vi "Projekt.vi"() -> ()   [LabVIEW 2022 SP3]
doc: "Use this template to build a standard state machine design pattern. Each state executes code and determines which state to transition to. Contrast this design pattern with the User Interface Event Handler pattern, in which code executes in response to user actions. Contrast this design pattern also with the Queued Message Handler pattern, in which each message handling code can queue zero or more new messages.\nNote: This template does not contain the most recent programming guidelines recommended by National Instruments. For a complete, project-based implementation of the Standard State Machine pattern, use the Create Project dialog box instead of this template."
uses:
  Projekt.ctt
  <vilib>/DAQmx/write.llb/DAQmx Write (Digital 1D Bool 1Chan 1Samp).vi
  <vilib>/DAQmx/create/channels.llb/DAQmx Create Channel (DO-Digital Output).vi
  <vilib>/DAQmx/create/channels.llb/DAQmx Create Channel (AI-Voltage-Basic).vi
  <vilib>/DAQmx/create/channels.llb/DAQmx Create Channel (DI-Digital Input).vi
  <vilib>/DAQmx/read.llb/DAQmx Read (Analog DBL 1Chan 1Samp).vi
  <vilib>/DAQmx/read.llb/DAQmx Read (Digital 1D Bool 1Chan 1Samp).vi
panel:
  in  "Buttons":enum32{"Force", "Mass", "Starting height"}(radio)
  in  "LED":tag="Dev3/port0/line0:5"
  in  "Knob":tag="Dev3/ai1"
  in  "Buttons":tag="Dev3/port1/line0:2"
  out "Max S [m]":dbl
  in  "Starting height [m]":dbl
  out "XY Graph":cluster{ext[], ext[]}(graph)
  out "Max H [m]":dbl
  out "V [m/s]":dbl
  in  "Mass [kg]":dbl
  in  "Stop":bool
  in  "Force [n]":dbl
  in  "Angle":dbl(knob) min=0.0 max=90.0 scale=0.0..90.0
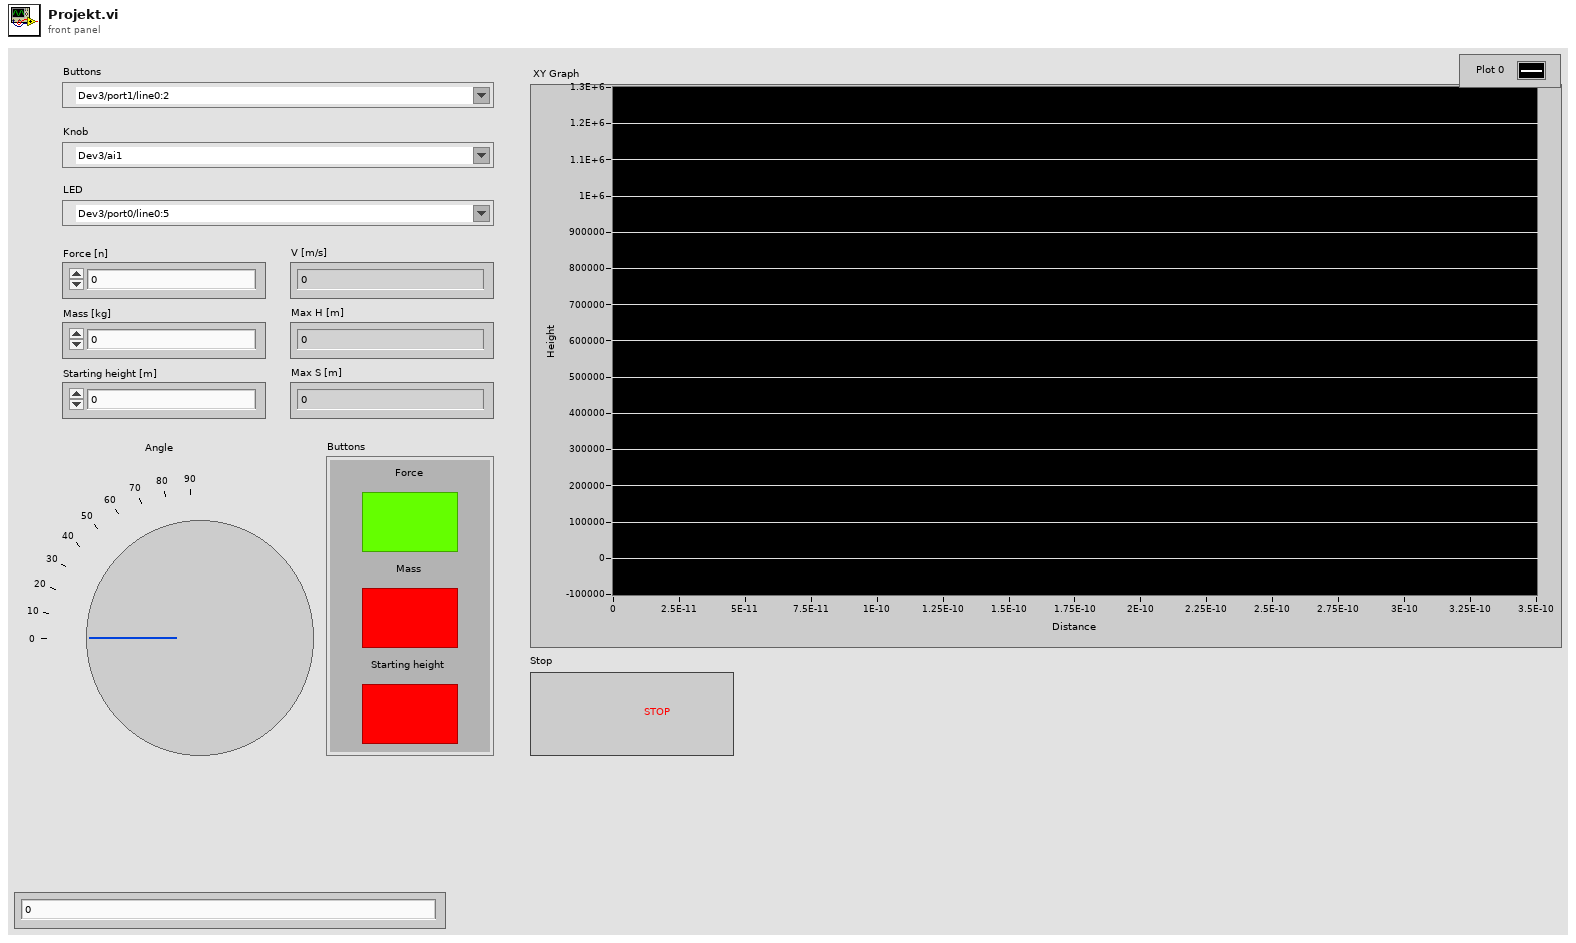
[diagram p1: front panel]
types:
  T1 = typedef "Projekt.ctt" = enum16{"Initialize", "Read", "Simulate", "Stop"}
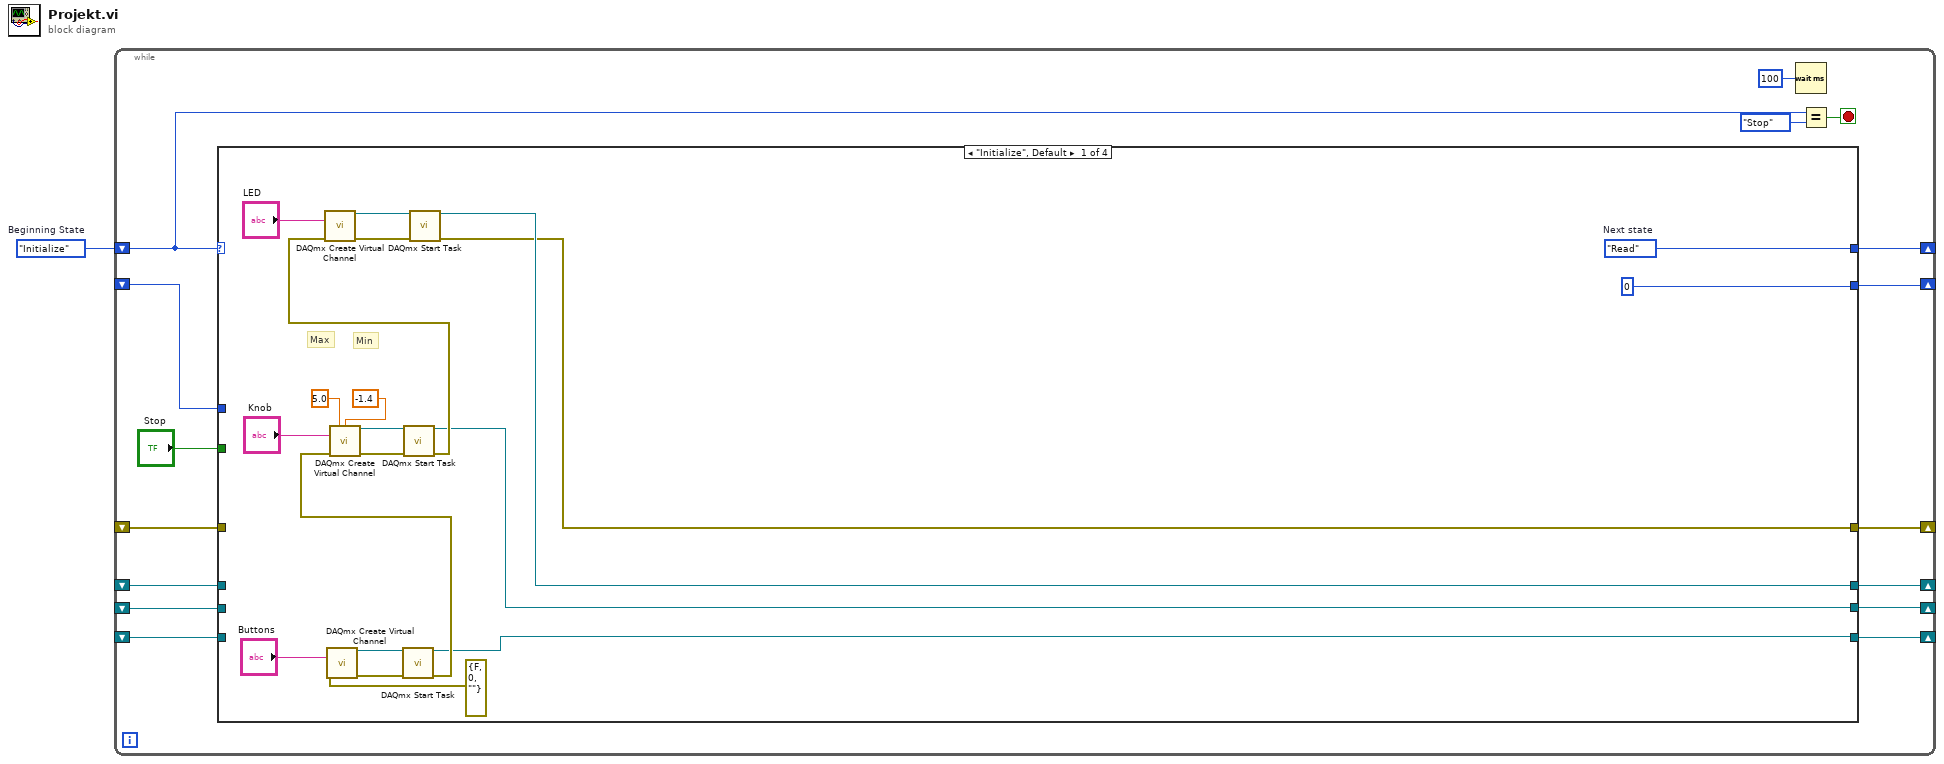
[diagram p0: block diagram]
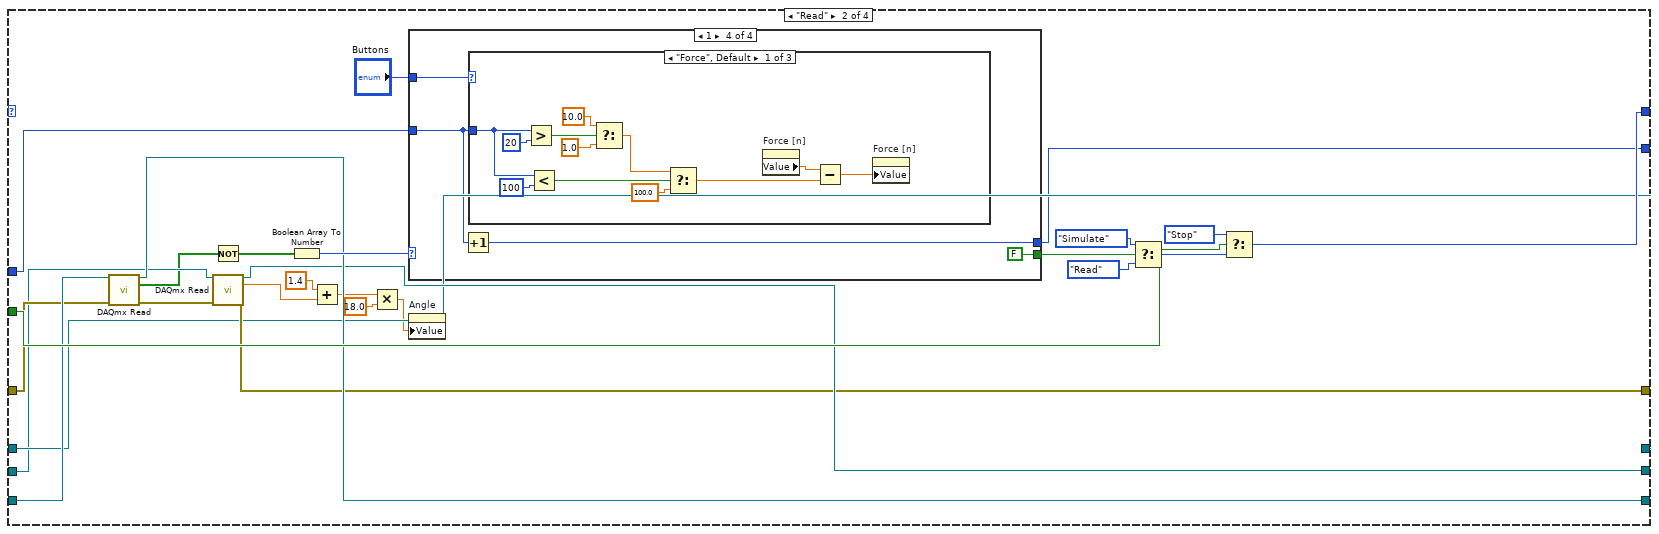
[diagram p2: hidden frame]
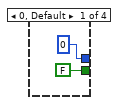
[diagram p3: hidden frame]
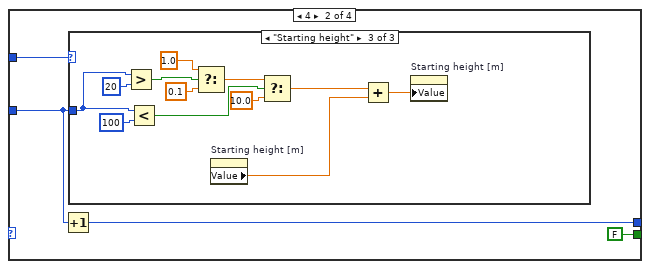
[diagram p4: hidden frame]
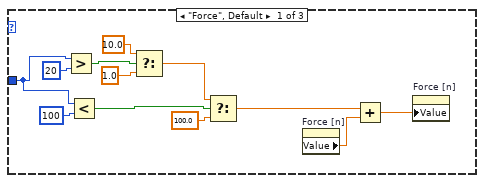
[diagram p5: hidden frame]
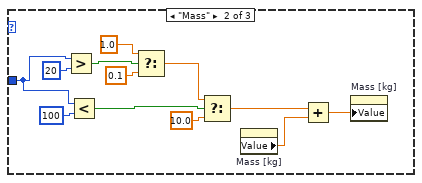
[diagram p6: hidden frame]
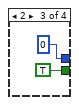
[diagram p7: hidden frame]
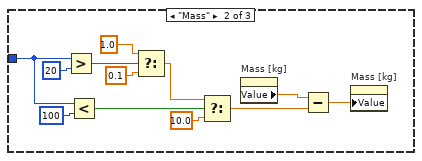
[diagram p8: hidden frame]
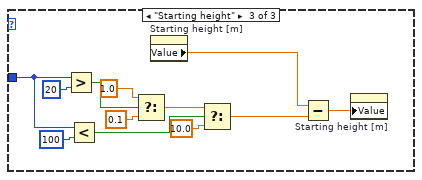
[diagram p9: hidden frame]
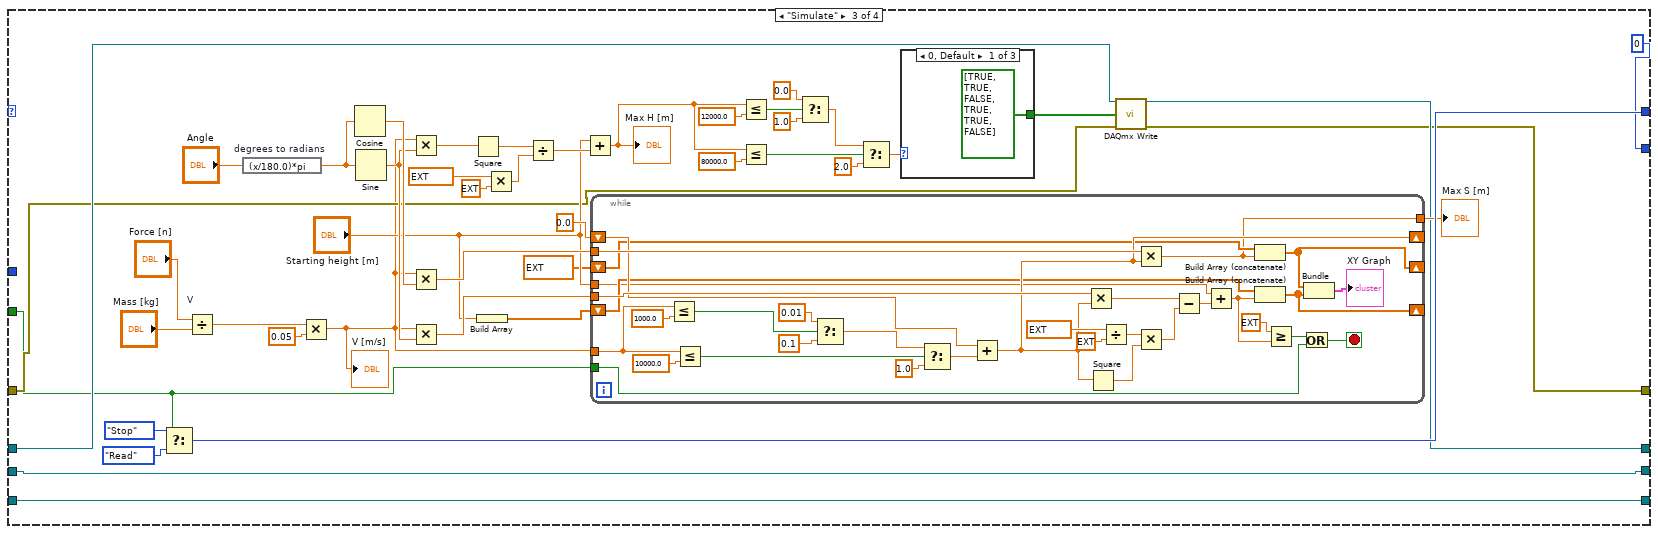
[diagram p10: hidden frame]
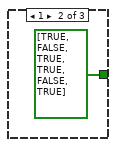
[diagram p11: hidden frame]
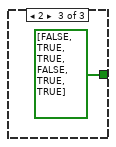
[diagram p12: hidden frame]
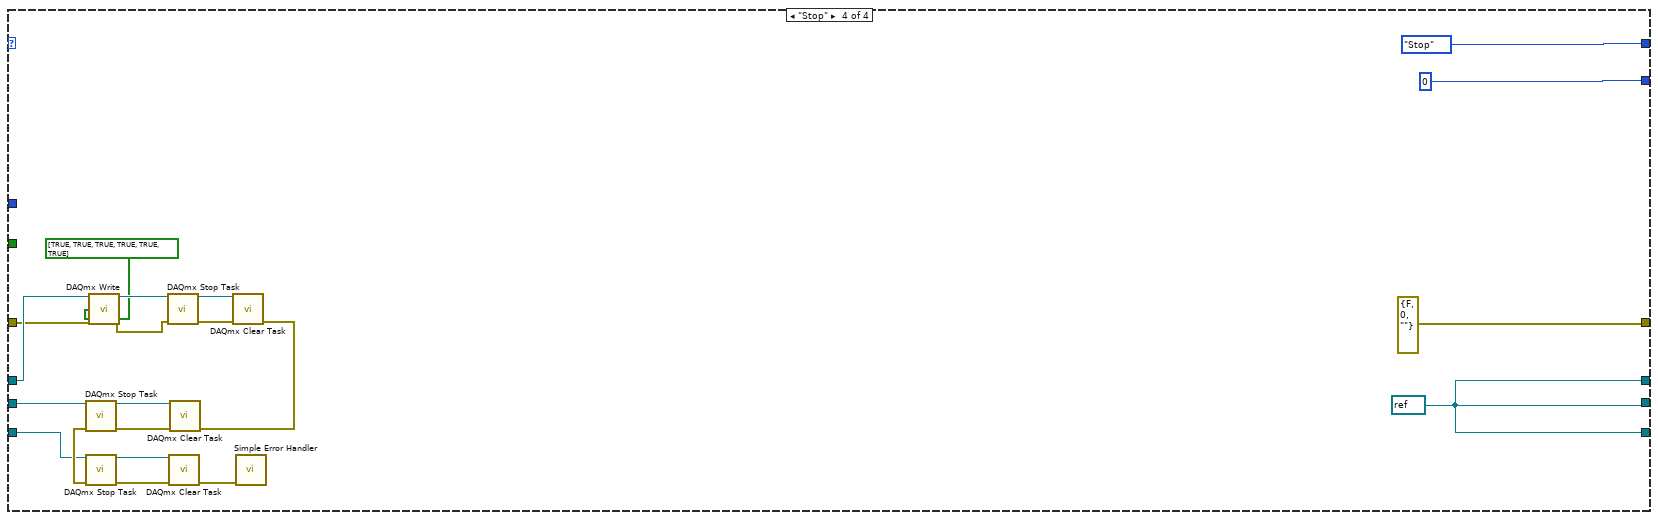
[diagram p13: hidden frame]
diagram:
  w1 = Projekt.ctt."Initialize"  # Beginning State
  n1 = while {
    shift-right: [w14] -> _
    shift-left: w1 -> [w15]
    shift-right: [w11] -> _
    shift-left: _ -> [w5]
    shift-right: [w10] -> _
    shift-left: _ -> [w6]
    shift-right: [w8] -> _
    shift-left: _ -> [w7]
    shift-right: [w9] -> _
    shift-left: _ -> [w4]
    shift-right: [w3] -> _
    shift-left: _ -> [w2]
    stop <- w17 stop-if-true
    n2 = case shown="\"Initialize\", Default" w15 {
      tunnel: [w18 w57 w178 Projekt.ctt."Stop" ("Next State")] -> w14
      tunnel: "Stop" -> [_ w56 w150 _]
      tunnel: w5 -> [_ w55 w168 w237]
      tunnel: [w25 w54 w168 w234] -> w11
      tunnel: [w24 w53 w167 w234] -> w10
      tunnel: [w23 w50 w154 w234] -> w8
      tunnel: [w22 w52 w153 errorcluster {"status"=FALSE, "code"=0, "source"=""} ("error constant")] -> w9
      tunnel: w4 -> [_ w51 w165 w231]
      tunnel: w7 -> [_ w50 w166 w232]
      tunnel: w6 -> [_ w49 w167 w236]
      tunnel: [0 w48 0 0] -> w3
      tunnel: w2 -> [_ w47 _ _]
      frame "Initialize", Default {
        w18 = Projekt.ctt."Read"  # Next state
        # "Max"
        # "Min"
        n3 = call-poly <vilib>:"DAQmx Create Virtual Channel.vi"("lines"="Buttons", "error in"=errorcluster {"status"=FALSE, "code"=0, "source"=""} ("error constant")) -> ("task out"=w37:refnum<k21>, "error out"=w36:errorcluster)  [unwired: 12 in]
        n4 = call <vilib>:"DAQmx Start Task.vi"("task/channels in"=w37, "error in"=w36) -> ("task out"=w25:refnum<k21>, "error out"=w30:errorcluster)  [unwired: 12 in]
        n5 = call-poly <vilib>:"DAQmx Create Virtual Channel.vi"("maximum value"=5.0, "minimum value"=-1.4, "physical channels"="Knob", "error in"=w30) -> ("task out"=w35:refnum<k21>, "error out"=w34:errorcluster)  [unwired: 10 in]
        n6 = call <vilib>:"DAQmx Start Task.vi"("task/channels in"=w35, "error in"=w34) -> ("task out"=w24:refnum<k21>, "error out"=w29:errorcluster)  [unwired: 12 in]
        n7 = call-poly <vilib>:"DAQmx Create Virtual Channel.vi"("lines"="LED", "error in"=w29) -> ("task out"=w33:refnum<k21>, "error out"=w32:errorcluster)  [unwired: 12 in]
        n8 = call <vilib>:"DAQmx Start Task.vi"("task/channels in"=w33, "error in"=w32) -> ("task out"=w23:refnum<k21>, "error out"=w22:errorcluster)  [unwired: 12 in]
      }
      frame "Read" {
        n9 = call-poly <vilib>:"DAQmx Read.vi"("task/channels in"=w55, "error in"=w51) -> ("task out"=w54:refnum<k21>, "data"=w42:bool[], "error out"=w63:errorcluster)  [unwired: 11 in]
        n10 = Not(x=w42) -> (.not. x?=w41:bool[])
        n11 = call-poly <vilib>:"DAQmx Read.vi"("task/channels in"=w49, "error in"=w63) -> ("task out"=w53:refnum<k21>, "data"=w45:dbl, "error out"=w52:errorcluster)  [unwired: 11 in]
        n12 = Boolean Array To Number(Boolean array=w41) -> (number=w60:u32)
        n13 = Add(x=1.4, y=w45) -> (x+y=w43:dbl)
        n14 = Multiply(x=w43, y=18.0) -> (x*y=w46:dbl)
        n15 = case shown="1" w60 {
          tunnel: "Buttons" -> [_ w69 _ w108]
          tunnel: [FALSE FALSE TRUE FALSE] -> w59
          tunnel: [0 w67 0 w109] -> w48
          tunnel: w47 -> [_ w66 _ w110]
          frame 0, Default {
          }
          frame 4 {
            n16 = Increment(x=w66) -> (x+1=w67:i32)
            n17 = case shown="\"Starting height\"" w69 {
              tunnel: w66 -> [w76 w85 w96]
              frame "Force", Default {
                n18 = Greater?(x=w76, y=20) -> (0:w80:bool)
                n19 = Less?(x=w76, y=100) -> (x < y?=w74:bool)
                n20 = Select(t=10.0, s=w80, f=1.0) -> (s? t:f=w77:dbl)
                n21 = Select(t=w77, s=w74, f=100.0) -> (s? t:f=w72:dbl)
                n22 = property on="Force [n]" class="DigNum (strict)"() -> ("Value"=w71:dbl)  [unwired: 2 in, 2 out]
                n23 = Add(x=w72, y=w71) -> (x+y=w70:dbl)
                n24 = property on="Force [n]" class="DigNum (strict)"("Value"=w70) -> ()  [unwired: 2 in, 2 out]
              }
              frame "Mass" {
                n25 = Greater?(x=w85, y=20) -> (0:w92:bool)
                n26 = Less?(x=w85, y=100) -> (x < y?=w87:bool)
                n27 = Select(t=1.0, s=w92, f=0.1) -> (s? t:f=w89:dbl)
                n28 = Select(t=w89, s=w87, f=10.0) -> (s? t:f=w84:dbl)
                n29 = property on="Mass [kg]" class="DigNum (strict)"() -> ("Value"=w83:dbl)  [unwired: 2 in, 2 out]
                n30 = Add(x=w84, y=w83) -> (x+y=w82:dbl)
                n31 = property on="Mass [kg]" class="DigNum (strict)"("Value"=w82) -> ()  [unwired: 2 in, 2 out]
              }
              frame "Starting height" {
                n32 = Greater?(x=w96, y=20) -> (0:w104:bool)
                n33 = Less?(x=w96, y=100) -> (x < y?=w99:bool)
                n34 = Select(t=1.0, s=w104, f=0.1) -> (s? t:f=w101:dbl)
                n35 = property on="Starting height [m]" class="DigNum (strict)"() -> ("Value"=w95:dbl)  [unwired: 2 in, 2 out]
                n36 = Select(t=w101, s=w99, f=10.0) -> (s? t:f=w97:dbl)
                n37 = Add(x=w97, y=w95) -> (x+y=w94:dbl)
                n38 = property on="Starting height [m]" class="DigNum (strict)"("Value"=w94) -> ()  [unwired: 2 in, 2 out]
              }
            }
          }
          frame 2 {
          }
          frame 1 {
            n39 = Increment(x=w110) -> (x+1=w109:i32)
            n40 = case shown="\"Force\", Default" w108 {
              tunnel: w110 -> [w113 w127 w138]
              frame "Force", Default {
                n41 = Greater?(x=w113, y=20) -> (0:w120:bool)
                n42 = Less?(x=w113, y=100) -> (x < y?=w115:bool)
                n43 = Select(t=10.0, s=w120, f=1.0) -> (s? t:f=w117:dbl)
                n44 = Select(t=w117, s=w115, f=100.0) -> (s? t:f=w112:dbl)
                n45 = property on="Force [n]" class="DigNum (strict)"() -> ("Value"=w123:dbl)  [unwired: 2 in, 2 out]
                n46 = Subtract(x=w123, y=w112) -> (x-y=w122:dbl)
                n47 = property on="Force [n]" class="DigNum (strict)"("Value"=w122) -> ()  [unwired: 2 in, 2 out]
              }
              frame "Mass" {
                n48 = Greater?(x=w127, y=20) -> (0:w134:bool)
                n49 = Less?(x=w127, y=100) -> (x < y?=w129:bool)
                n50 = Select(t=1.0, s=w134, f=0.1) -> (s? t:f=w131:dbl)
                n51 = Select(t=w131, s=w129, f=10.0) -> (s? t:f=w124:dbl)
                n52 = property on="Mass [kg]" class="DigNum (strict)"() -> ("Value"=w126:dbl)  [unwired: 2 in, 2 out]
                n53 = Subtract(x=w126, y=w124) -> (x-y=w125:dbl)
                n54 = property on="Mass [kg]" class="DigNum (strict)"("Value"=w125) -> ()  [unwired: 2 in, 2 out]
              }
              frame "Starting height" {
                n55 = Greater?(x=w138, y=20) -> (0:w146:bool)
                n56 = Less?(x=w138, y=100) -> (x < y?=w141:bool)
                n57 = Select(t=1.0, s=w146, f=0.1) -> (s? t:f=w143:dbl)
                n58 = property on="Starting height [m]" class="DigNum (strict)"() -> ("Value"=w137:dbl)  [unwired: 2 in, 2 out]
                n59 = Select(t=w143, s=w141, f=10.0) -> (s? t:f=w139:dbl)
                n60 = Subtract(x=w137, y=w139) -> (x-y=w136:dbl)
                n61 = property on="Starting height [m]" class="DigNum (strict)"("Value"=w136) -> ()  [unwired: 2 in, 2 out]
              }
            }
          }
        }
        n62 = property on="Angle" class="Knob (strict)"("Value"=w46) -> ()  [unwired: 2 in, 2 out]
        n63 = Select(t=Projekt.ctt."Simulate" ("States"), s=w59, f=Projekt.ctt."Read" ("States")) -> (s? t:f=w61:T1)
        n64 = Select(t=Projekt.ctt."Stop" ("States"), s=w56, f=w61) -> (s? t:f=w57:T1)
      }
      frame "Simulate" {
        n65 = Select(t=Projekt.ctt."Stop" ("States"), s=w150, f=Projekt.ctt."Read" ("States")) -> (s? t:f=w178:T1)
        n66 = Divide "V"(x="Force [n]", y="Mass [kg]") -> (x/y=w175:dbl)
        n67 = expression code="(x/180.0)*pi" "degrees to radians"("Angle") -> (w185:dbl)
        n68 = Multiply(x=w175, y=0.05) -> (x*y=w149:dbl)
        "V [m/s]" <- w149
        n69 = Cosine(x=w185) -> (cos(x)=w184:dbl)
        n70 = Sine(x=w185) -> (sin(x)=w182:dbl)
        n71 = Multiply(x=w149, y=w182) -> (x*y=w177:dbl)
        n72 = Multiply(x=w149, y=w184) -> (x*y=w183:dbl)
        n73 = Multiply(x=w149, y=w182) -> (x*y=w181:dbl)
        n74 = Square(x=w177) -> (x^2=w176:dbl)
        n75 = Build Array("Starting height [m]") -> (w171:dbl[])
        n76 = Multiply(x=ext 9.80665, y=ext 2.0) -> (x*y=w187:ext)
        n77 = Divide(x=w176, y=w187) -> (x/y=w173:ext)
        n78 = Add(x="Starting height [m]", y=w173) -> (x+y=w152:ext)
        "Max H [m]" <- w152
        n79 = while {
          tunnel: w183 -> [w227]
          tunnel: w181 -> [w226]
          shift-right: [w218] -> _
          shift-left: 0.0 ("x") -> [w223]
          shift-right: [w213] -> _
          shift-left: ext[] [0.0] ("array") -> [w215]
          shift-right: [w212] -> _
          shift-left: w171 -> [w216]
          tunnel: "Starting height [m]" -> [w211]
          tunnel: [w208] -> w169
          tunnel: w150 -> [w206]
          tunnel: w149 -> [w199]
          stop <- w205 stop-if-true
          n80 = Less Or Equal?(x=w199, y=1000.0) -> (x <= y?=w200:bool)
          n81 = Less Or Equal?(x=w199, y=10000.0) -> (x <= y?=w197:bool)
          n82 = Select(t=0.01 ("y"), s=w200, f=0.1) -> (s? t:f=w202:dbl)
          n83 = Select(t=w202, s=w197, f=1.0) -> (s? t:f=w195:dbl)
          n84 = Add(x=w223, y=w195) -> (x+y=w218:dbl)
          n85 = Multiply(x=w226, y=w218) -> (x*y=w220:dbl)
          n86 = Square(x=w218) -> (x^2=w222:dbl)
          n87 = Divide(x=ext 9.80665, y=ext 2.0) -> (x/y=w221:ext)
          n88 = Multiply(x=w227, y=w218) -> (x*y=w208:dbl)
          n89 = Multiply(x=w221, y=w222) -> (x*y=w219:ext)
          n90 = Subtract(x=w220, y=w219) -> (x-y=w210:ext)
          n91 = Add(x=w211, y=w210) -> (x+y=w209:ext)
          n92 = Build Array (concatenate)(w215, w208) -> (w213:ext[])
          n93 = Build Array (concatenate)(w216, w209) -> (w212:ext[])
          n94 = Greater Or Equal?(x=ext 0.0, y=w209) -> (x >= y?=w207:bool)
          n95 = Or(x=w207, y=w206) -> (x .or. y?=w205:bool)
          n96 = Bundle(w213, w212) -> (→"XY Graph":cluster{ext[], ext[]})  [unwired: 1 in]
        }
        "Max S [m]" <- w169
        n97 = Less Or Equal?(x=w152, y=12000.0) -> (x <= y?=w163:bool)
        n98 = Less Or Equal?(x=w152, y=80000.0) -> (x <= y?=w159:bool)
        n99 = Select(t=0.0, s=w163, f=1.0) -> (s? t:f=w157:dbl)
        n100 = Select(t=w157, s=w159, f=2.0) -> (s? t:f=w156:dbl)
        n101 = case shown="0, Default" w156 {
          tunnel: [bool[] [TRUE, TRUE, FALSE, TRUE, TRUE, FALSE] ("data") bool[] [TRUE, FALSE, TRUE, TRUE, FALSE, TRUE] ("data") bool[] [FALSE, TRUE, TRUE, FALSE, TRUE, TRUE] ("data")] -> w155
          frame 0, Default {
          }
          frame 1 {
          }
          frame 2 {
          }
        }
        n102 = call-poly <vilib>:"DAQmx Write.vi"("task/channels in"=w166, "data"=w155, "error in"=w165) -> ("task out"=w154:refnum<k21>, "error out"=w153:errorcluster)  [unwired: 10 in, 1 out]
      }
      frame "Stop" {
        w234 = refnum<k21> refnum ("task out")
        n103 = call-poly <vilib>:"DAQmx Write.vi"("task/channels in"=w232, "data"=bool[] [TRUE, TRUE, TRUE, TRUE, TRUE, TRUE], "error in"=w231) -> ("task out"=w229:refnum<k21>, "error out"=w230:errorcluster)  [unwired: 10 in, 1 out]
        n104 = call <vilib>:"DAQmx Stop Task.vi"("task/channels in"=w229, "error in"=w230) -> ("task out"=w244:refnum<k21>, "error out"=w243:errorcluster)  [unwired: 12 in]
        n105 = call <vilib>:"DAQmx Clear Task.vi"("task in"=w244, "error in"=w243) -> ("error out"=w242:errorcluster)  [unwired: 13 in]
        n106 = call <vilib>:"DAQmx Stop Task.vi"("task/channels in"=w236, "error in"=w242) -> ("task out"=w245:refnum<k21>, "error out"=w241:errorcluster)  [unwired: 12 in]
        n107 = call <vilib>:"DAQmx Clear Task.vi"("task in"=w245, "error in"=w241) -> ("error out"=w240:errorcluster)  [unwired: 13 in]
        n108 = call <vilib>:"DAQmx Stop Task.vi"("task/channels in"=w237, "error in"=w240) -> ("task out"=w246:refnum<k21>, "error out"=w239:errorcluster)  [unwired: 12 in]
        n109 = call <vilib>:"DAQmx Clear Task.vi"("task in"=w246, "error in"=w239) -> ("error out"=w238:errorcluster)  [unwired: 13 in]
        n110 = call <vilib>:"Simple Error Handler.vi"("error in (no error)"=w238) -> ()  [unwired: 4 in, 5 out]
      }
    }
    n111 = Wait (ms)(milliseconds to wait=u32 100) -> ()  [unwired: 1 out]
    n112 = Equal?(x=w15, y=Projekt.ctt."Stop" ("States")) -> (x = y?=w17:bool)
  }
